vi "SLL DE Compare Continuous AI Channel Enum and MAX Channel.vi"(8 "error in (no error)":errorcluster, 11 "Analog Input Channels":refnum<k21>[](array[refnum])) -> (0 "error out":errorcluster, 3 "Channels Out":refnum<k21>[](array[refnum]), 5 "Pass?":bool)   [LabVIEW 2013]
doc: "This VI will check and seperate all Analog Inputs listed in enum form global Channel list\n\nCreated by Yogesh Redemptor, \nCopyright © 2008, Soliton Technologies.\nAll rights reserved."
uses:
  Controls/SLL DE List of Analog Inputs.ctl
panel:
  in  "List of Analog Inputs":T1
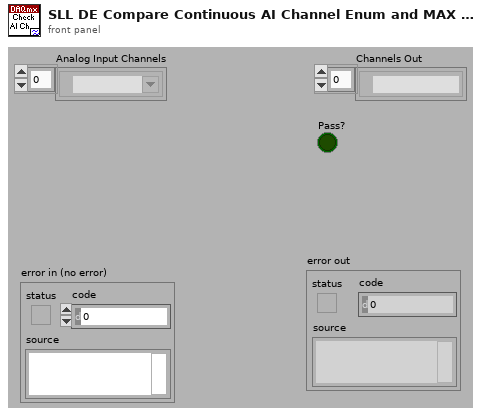
[diagram p1: front panel]
types:
  T1 = typedef "SLL DE List of Analog Inputs.ctl" = enum16{"None"}
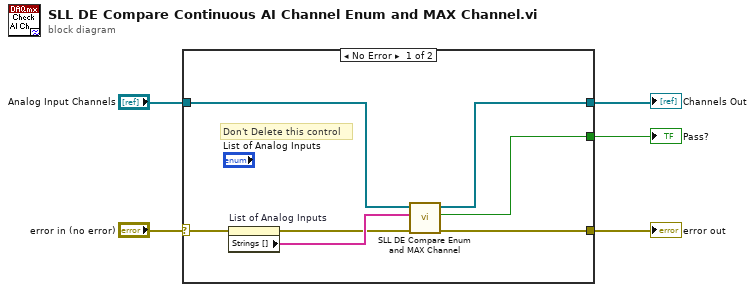
[diagram p0: block diagram]
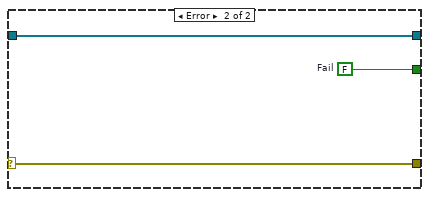
[diagram p2: hidden frame]
diagram:
  n1 = case shown="No Error" "error in (no error)" {
    selector: "error in (no error)" -> [w12 w15]
    tunnel: [w8 w15] -> w4
    tunnel: "Analog Input Channels" -> [w10 w14]
    tunnel: [w7 w13] -> w2
    tunnel: [w6 w14] -> w1
    frame No Error {
      # "Don't Delete this control"
      n2 = property on="List of Analog Inputs" class="Enum (strict)"(error in=w12) -> (error out=w9:errorcluster, "Strings []"=w11:string[])  [unwired: 1 in, 1 out]
      n3 = call "SLL DE Compare Enum and MAX Channel.vi"("error in (no error)"=w9, "Strings []"=w11, "Channels In"=w10) -> ("error out"=w8:errorcluster, "Pass?"=w7:bool, "Channels Out"=w6:refnum<k21>[])  [unwired: 6 in]
    }
    frame Error {
      w13 = FALSE  # Fail
    }
  }
  "error out" <- w4
  "Pass?" <- w2
  "Channels Out" <- w1
